vi "ERIO RT Main.vi"() -> ()   [LabVIEW 2017]
doc: "The top-level Real-Time VI for the RIO Eval Kit.\n\nThis VI runs through multiple stages. Each stage demonstrates different features of the RIO Eval Kit. The program uses a \"Queued Message Handler\" architecture. The top loop reads and writes information to and from the FPGA. That information is sent to the bottom through a queue. The information being transfered includes both the data and the type of message being sent. The bottom loop then handles displaying the appropriate information on the LCD. \n\nThe EEI IoT update to this program expands the conveyor simulation. As the encoder is moved the simulation goes through stages 1-3. When the end of 3 is met then it goes through a shutdown and back to a process reset state. At any time a shutdown, from a local source or the remote supervisor UI will put it in a reset process state. Other functions are:\n- the right button will call for an E-STOP, which will terminate the RT program\n- Alarms for signal threshold reached\n- Notifications for stage transitions and shutdown\n- Signal capture of 800 samples when triggered. \n\nInteractions are enabled by NI SystemLink, the LabVIEW Cloud Toolkit for AWS, and the LabVIEW WebVI. \n\nORIGINAL CODE: \nBy: National Instruments\n NI LabVIEW RIO Evaluation Kit\n Code example \"5- Startup Application\"\n www.ni.com/embeddedsystems\n\nUPDATED CODE: Adds NI SystemLink and NI AWS LabVIEW Tookit functionality for demonstration. \nBy: James Tillett\n Endeavor Engineering Inc.\n www.endeavoreng.com"
uses:
  <vilib>/AWS Toolkit/Core/HTTP Request/Region.ctl
  LabVIEW/Real-Time/EmbeddedDisplay/Hitachi HD44780/Common/Control/screen size.ctl
  LabVIEW/Real-Time/EmbeddedDisplay/Hitachi HD44780/Common/Control/font configuration.ctl
  LabVIEW/Controls/ERIO Queue Data.ctl
  Class EEISysLink/EEISysLink.lvclass
  LabVIEW/Controls/ERIO AWS Toolkit Variables.ctl
  <vilib>/AWS Toolkit/SQS/Queue/Queue.lvclass
  <vilib>/AWS Toolkit/SNS/Phone Number/Phone Number.lvclass
  <vilib>/AWS Toolkit/S3/Bucket/Bucket.lvclass
  LabVIEW/Controls/ERIO RT State Variables.ctl
  LabVIEW/Controls/ERIO SystemStates.ctl
  LabVIEW/Controls/ERIO Worker Variables.ctl
  LabVIEW/Controls/ERIO Globals.vi
  <vilib>/FPGAPlugInAG/sbRIO-9637/niLvFpga_Open_sbRIO-9637.vi
  <vilib>/rvi/interface/common/dynamic/niFpgaDynamicAddResources.vi
  <vilib>/Utility/error.llb/Error Cluster From Error Code.vi
  <vilib>/rvi/errors/niLvFpgaAdjustHostInterfaceError.vi
  <vilib>/FPGAPlugInAG/Dynamic/niLvFpga_Close_Dynamic.vi
  <vilib>/rvi/interface/nirviOpenFPGA/nirviOpenFPGA.xnode
  FPGA Bitfiles/ERIOLabVIEW_IoTEx_FPGATarget_FPGA_TbyGp41NgaI.lvbitx
  <vilib>/rvi/interface/nirviReadWriteControl/nirviReadWriteControl.xnode
  <vilib>/rvi/interface/nirviCloseFPGA/nirviCloseFPGA.xnode
  LabVIEW/Real-Time/EmbeddedDisplay/Hitachi HD44780/Common/HD44780 Common.lvlib
  LabVIEW/Real-Time/EmbeddedDisplay/Hitachi HD44780/Host/HD44780 Host.lvlib
  <vilib>/rvi/interface/Simulation/niFpgaSimulationCallBeginRW.vi
  NiFpgaLv.dll
  <vilib>/AWS Toolkit/Core/HTTP Request/HTTP Request.lvclass
panel:
  out "error out":errorcluster
  in  "Secret Key":string="1234567890abcdefghijklmnopqrstuvwxyz09876543221"
  out "Access Key":string
  out "Region":T1=enum."us-west-2"
  out "Phone Number":string
  out "Enable SystemLink Signal Capture":bool=TRUE
  out "Last Triggered Signal Capture":waveform(dbl)(graph)
  out "Enable S3 TDMS Signal Capture":bool=TRUE
  out "Enable SQS Notification":bool=TRUE
  out "Enable SNS Stage Notification":bool=TRUE
  out "Enable SNS Alarm Notification":bool=TRUE
  out "State":string
  out "Loop Iterations":i32
  out "Last Signal Update":waveform(dbl)(graph)
  out "Alarm":bool
  out "Alarm Threshold":dbl=4.0 format="%.3g"
  out "Amplitude":dbl format="%.3f"
  # "Start by turning encoder right to kickoff first stage, and \ncontinue turning right to complete all three stages. Stop \nthe program at any time by pressing the right button (PB2)."
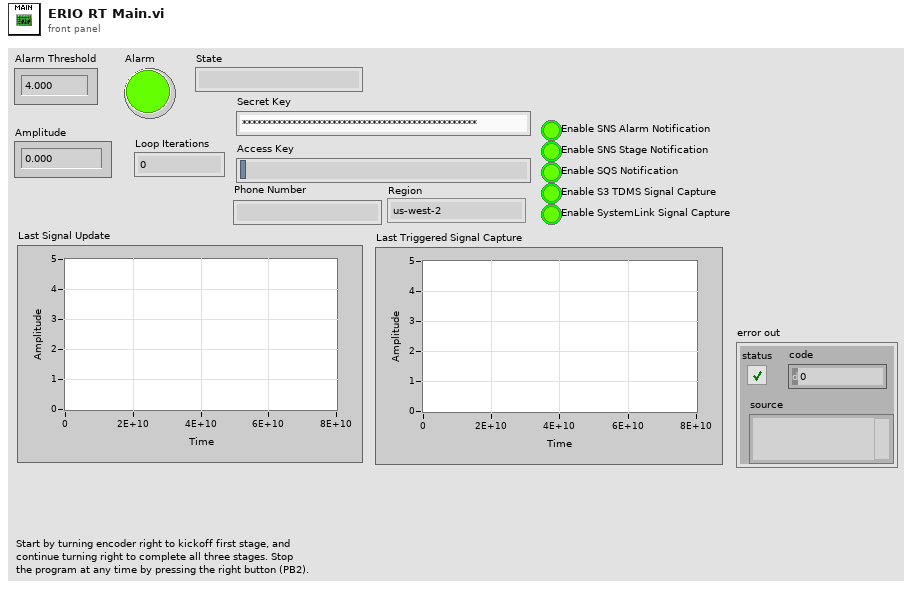
[diagram p1: front panel]
types:
  T1 = typedef "NI_AWS_Core.lvlib/HTTP Request.lvclass/Region.ctl" = enum16{"us-east-1", "us-east-2", "us-west-1", "us-west-2", "ap-northeast-1", "ap-northeast-2", "ap-southeast-1", "ap-southeast-2", "ca-central-1", "eu-central-1", "eu-west-1", "eu-west-2", "sa-east-1"}
  T2 = typedef "ERIO SystemStates.ctl" = enum16{"Shutdown", "E-STOP", "Reset Process", "Stage 1", "Stage 2", "Stage 3", "Alarm State"}
  T3 = typedef "ERIO RT State Variables.ctl" = cluster{"Position (local)":i16, "E-Stop":bool, "System State":T2, "FPGA Ref":refnum<k20>, "Previous Position (local)":i16, "Consumer Queue":refnum<queue>, "Worker Variables":T4, "Threshold Alarm":bool, "User Button":bool, "Last Signal Update":waveform(dbl)}
  T4 = typedef "ERIO Worker Variables.ctl" = cluster{"Signal Amplitude":dbl, "State":string, "Stage Percent Complete":dbl, "Alarm State":bool, "Capture Available":bool}
  T5 = typedef "ERIO AWS Toolkit Variables.ctl" = cluster{"SQS Queue":refnum<class "Queue.lvclass">, "SNS Phone Number":refnum<class "Phone Number.lvclass">, "S3 Bucket":refnum<class "Bucket.lvclass">, "SQS Init?":bool, "S3 Init?":bool, "SNS Init?":bool}
  T6 = typedef "ERIO Queue Data.ctl" = cluster{"Transition Requested":bool, "Current Pos > Previous?":bool, "Amplitude":dbl, "Stage Number":string}
  T7 = typedef "HD44780 Common.lvlib/font configuration.ctl" = enum8{"5x8 & 2 lines", "5x10 & 1 line", "5x8 & 1 line"}
  T8 = typedef "HD44780 Common.lvlib/screen size.ctl" = enum8{"8x1", "8x2", "12x4", "16x1", "16x2", "16x4", "20x1", "20x2", "20x4", "24x1", "24x2", "40x2", "40x4"}
  T9 = typedef "EEISysLink.lvclass/SL Tag Properties.ctl" = cluster{"Class Data Type":T10, "Name":string, "Description":string, "Interpolation Method":T11, "Unit of Measure":T12, "Maximum Interpolation":string, "Role":T13}
  T10 = typedef "EEISysLink.lvclass/SL Tag Data Type.ctl" = enum16{"Double", "Integer", "String", "Boolean", "Waveform"}
  T11 = typedef "EEISysLink.lvclass/SL Tag Interpolation Method.ctl" = enum16{"linear", "pilinear", "step"}
  T12 = typedef "EEISysLink.lvclass/SL Tag Unit of Measure.ctl" = enum16{"no units", "Second", "Hour", "Minute", "Day", "Year", "Month", "Week", "Foot", "Yard", "Meter", "Centimeter", "Inch", "Mile", "Nautical Mile", "Miles per Hour", "Meters per second", "Square meter", "Cubic meter", "Cubic centimeter", "Cubic inch", "Liter", "Gallon", "Gallons dry US", "Gallon UK", "Percent", "Revolutions per minute", "Revolution", "Degree angle", "Astronomical Unit", "Atom", "Atomic mass", "Bar", "Byte", "C (speed of light)", "Curie", "Decibel", "Electron Volt", "Ounce", "Knot", "G", "Grade", "Are", "Hectare", "Faraday", "Franklin", "Gilbert", "Erg", "Lambert", "Maxwell", "Gauss", "Electron mass", "Kilogram force", "Pound force", "Rad", "Centiradian", "Sphere", "Mach", "Fluid Ounces", "Fluid Ounces UK", "Fahrenheit", "Celsius", "Kelvin", "Rankine", "Gram", "Kilogram", "Pound", "Short/US Ton", "Long/UK ton", "Metric ton", "Mole", "Pounds per square inch", "Inches water column", "Torr", "Millitorr", "Millimeter mercury", "Inches mercury", "Bar (2)", "Atmosphere", "Pascal", "Watt", "kiloWatt", "Horsepower", "Kilowatt Hour", "British thermal units", "Millions of BTU", "Ampere", "Candela", "Radian", "Steradian", "Bit", "Hertz", "Newton", "Joule", "Coulomb", "Volt", "Farad", "Ohm", "Siemens", "Weber", "Tesla", "Henry", "Lumen", "Lux", "Becqueral", "Gray", "Sievert", "Katal", "Angstrom", "Light Year", "Parsec", "Point", "Pixel", "Dyne", "Kilogram force (2)", "Pound force (2)", "Rem", "Rutherford", "Roentgen"}
  T13 = typedef "EEISysLink.lvclass/SL Tag Type.ctl" = enum16{"All", "Supervisor", "Worker"}
  T14 = typedef "ERIO Supervisory Variables.ctl" = cluster{"Alarm Threshold":dbl, "Shutdown":bool, "Enable SNS Alarm":bool, "Enable SNS Stage Notification":bool, "Enable SQS Notification":bool, "Enable S3 TDMS Signal Capture":bool, "Enable SystemLink Signal Capture":bool, "Capture Signal":bool, "Server Update":bool, "AWS Access Key":string, "AWS Secret Key":string, "Phone Number":string, "Region":T1, "AWS SQS Queue":string, "AWS S3 Bucket":string}
  T15 = typedef "ERIO Alarm-Notifier Action.ctl" = enum16{"No Action", "Threshold Alarm", "Into Stage 1", "Into Stage 2", "Into Stage 3", "Into Shutdown", "Into Process Reset", "Into E-STOP", "User Button"}
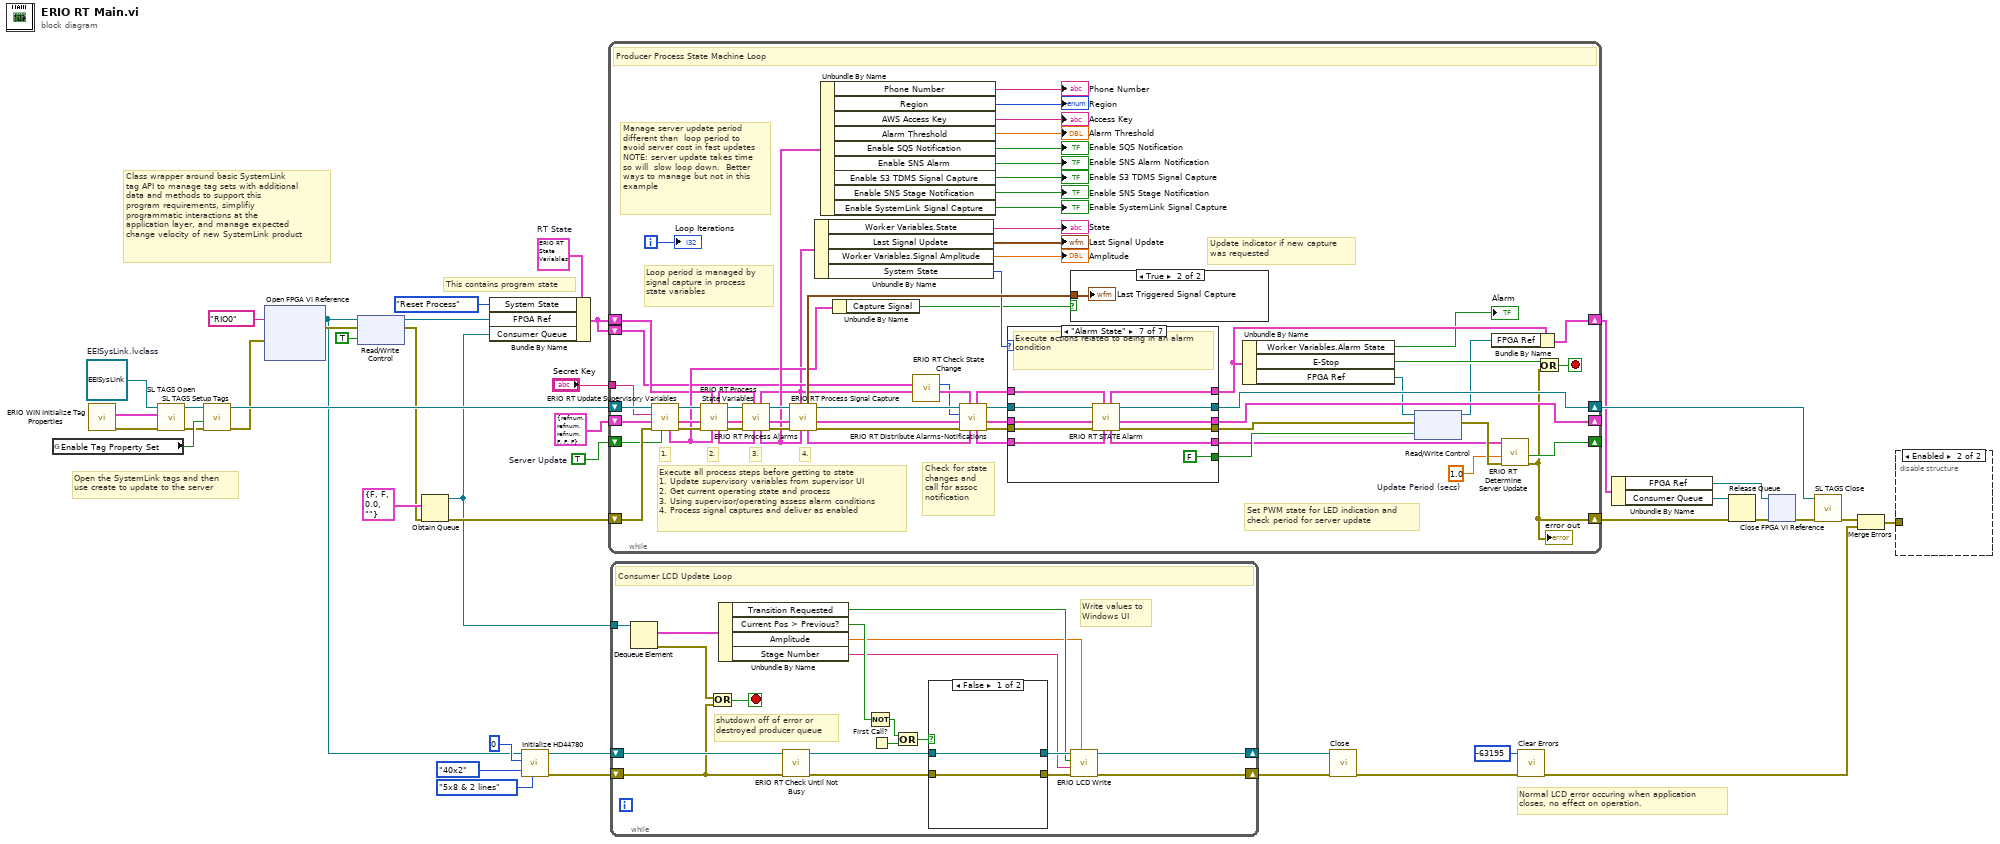
[diagram p0: block diagram]
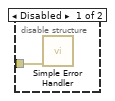
[diagram p2: hidden frame]
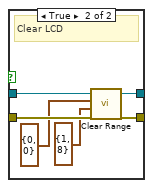
[diagram p3: hidden frame]
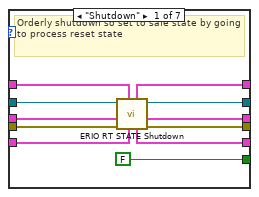
[diagram p5: hidden frame]
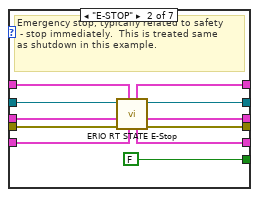
[diagram p6: hidden frame]
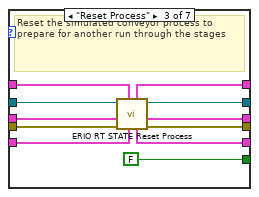
[diagram p7: hidden frame]
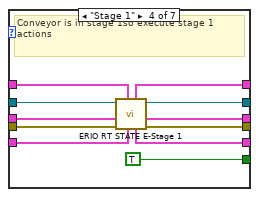
[diagram p8: hidden frame]
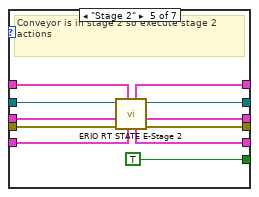
[diagram p9: hidden frame]
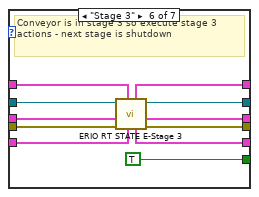
[diagram p10: hidden frame]
diagram:
  w16 = T3 {"Position (local)"=0, "E-Stop"=FALSE, "System State"=enum."Shutdown", "FPGA Ref"=refnum, "Previous Position (local)"=2, "Consumer Queue"=refnum, "Worker Variables"={"Signal Amplitude"=0.0, "State"="", "Stage Percent Complete"=0.0, "Alarm State"=FALSE, "Capture Available"=FALSE}, "Threshold Alarm"=FALSE, "User Button"=FALSE, "Last Signal Update"={"t0"=timestamp(0 s since 1904-01-01), "dt"=1.0, "Y"=[]}}  # RT State
  w20 = TRUE  # Server Update
  w23 = refnum<class "EEISysLink.lvclass"> refnum  # EEISysLink.lvclass
  # "Class wrapper around basic SystemLink\ntag API to manage tag sets with additional\ndata and methods to support this \nprogram requirements, simplifiy\nprogrammatic interactions at the \napplication layer, and manage expected\nchange velocity of new SystemLink product"
  # "This contains program state"
  # "Open the SystemLink tags and then\nuse create to update to the server"
  # "Normal LCD error occuring when application\ncloses, no effect on operation."
  n1 = global read "ERIO Globals.vi" "Enable Tag Property Set"() -> (w26:bool)
  n2 = call "ERIO WIN Initialize Tag Properties.vi"() -> ("error out"=w25:errorcluster, "Tag Properties"=w2:T9[])  [unwired: 9 in, 1 out]
  n3 = call-dynamic "SL TAGS Open.vi"("error in (no error)"=w25, "Tag Properties"=w2, "EEISysLink in"=w23) -> ("error out"=w24:errorcluster, "EEISysLink out"=w1:refnum<class "EEISysLink.lvclass">)  [unwired: 7 in]
  n4 = call-dynamic "SL TAGS Setup Tags.vi"("error in (no error)"=w24, "Set  Properties? (F)"=w26, "EEISysLink in"=w1) -> ("error out"=w22:errorcluster, "EEISysLink out"=w28:refnum<class "EEISysLink.lvclass">)  [unwired: 7 in]
  n5 = xnode ("Open FPGA VI Reference")("error in"=w22, "resource name"=tag "RIO0") -> ("FPGA VI Reference Out"=w4:refnum<k20>, "error out"=w7:errorcluster)
  n6 = xnode "Read/Write Control"("FPGA VI Reference In"=w4, "error in"=w7, "Reset"=TRUE) -> ("FPGA VI Reference Out"=w9:refnum<k20>, "error out"=w6:errorcluster)
  n7 = Obtain Queue(element data type=T6 {"Transition Requested"=FALSE, "Current Pos > Previous?"=FALSE, "Amplitude"=0.0, "Stage Number"=""} ("output to queue"), error in (no error)=w6) -> (queue out=w14:refnum<queue>, error out=w32:errorcluster)  [unwired: 3 in, 1 out]
  n8 = Bundle By Name(cluster=w16, "System State"=ERIO_SystemStates."Reset Process", "FPGA Ref"=w9, "Consumer Queue"=w14) -> (w5:T3)
  n9 = call "Initialize HD44780.vi"("font configuration (5x8 & 2 lines)"=font_configuration."5x8 & 2 lines", "screen size"=screen_size."40x2", "device index"=i8 0, "FPGA VI Reference in"=w4) -> ("error out"=w36:errorcluster, "LCD out"=w37:refnum<class "Character LCD.lvclass">)  [unwired: 6 in]
  n10 = while {
    shift-right: [w43] -> w42
    shift-left: w32 -> [w96]
    shift-right: [w73] -> w12
    shift-left: w5 -> [w62]
    shift-right: [w78] -> w18
    shift-left: w28 -> [w103]
    shift-right: [w77] -> _
    shift-left: T5 {"SQS Queue"=refnum, "SNS Phone Number"=refnum, "S3 Bucket"=refnum, "SQS Init?"=FALSE, "S3 Init?"=FALSE, "SNS Init?"=FALSE} ("AWS Variables In") -> [w102]
    shift-right: [w83] -> _
    shift-left: w20 -> [w84]
    shift-left: w5 -> [w61]
    tunnel: "Secret Key" -> [w45]
    i -> [w106]
    stop <- w97 stop-if-true
    w81 = 1.0  # Update Period (secs)
    # "4."
    # "3."
    # "2."
    # "1."
    # "Check for state\nchanges and\ncall for assoc\nnotification"
    # "Loop period is managed by\nsignal capture in process\nstate variables"
    # "Update indicator if new capture\nwas requested"
    # "Manage server update period\ndifferent than  loop period to\navoid server cost in fast updates\nNOTE: server update takes time\nso will  slow loop down.  Better\nways to manage but not in this\nexample"
    # "Set PWM state for LED indication and\ncheck period for server update"
    # "Execute all process steps before getting to state\n1. Update supervisory variables from supervisor UI\n2. Get current operating state and process\n3. Using supervisor/operating assess alarm conditions\n4. Process signal captures and deliver as enabled"
    # "Producer Process State Machine Loop"
    n11 = call "ERIO RT Update Supervisory Variables.vi"("Server Update"=w84, "error in (no error)"=w96, "AWS Variables In"=w102, "Secret Key"=w45, "EEISysLink.lvclass In"=w103) -> ("error out"=w104:errorcluster, "AWS Variables Out"=w101:T5, "EEISysLink.lvclass Out"=w105:refnum<class "EEISysLink.lvclass">, "Supervisory Variables"=w64:T14)  [unwired: 3 in]
    n12 = call "ERIO RT Process State Variables.vi"("Supervisory Variables In"=w64, "RT State In"=w62, "error in (no error)"=w104, "AWS Variables In"=w101, "EEISysLink.lvclass In"=w105) -> ("error out"=w98:errorcluster, "AWS Variables Out"=w99:T5, "EEISysLink.lvclass Out"=w100:refnum<class "EEISysLink.lvclass">, "Supervisory Variables Out"=w67:T14, "RT State Out"=w91:T3)  [unwired: 2 in]
    n13 = call "ERIO RT Process Alarms.vi"("Supervisory Variables In"=w67, "RT State In"=w91, "error in (no error)"=w98, "AWS Variables In"=w99, "EEISysLink.lvclass In"=w100) -> ("error out"=w92:errorcluster, "AWS Variables Out"=w93:T5, "EEISysLink.lvclass Out"=w94:refnum<class "EEISysLink.lvclass">, "Supervisory Variables Out"=w66:T14, "RT State Out"=w60:T3)  [unwired: 2 in]
    n14 = call "ERIO RT Process Signal Capture.vi"("Supervisory Variables In"=w66, "RT State"=w60, "error in (no error)"=w92, "AWS Variables In"=w93, "EEISysLink.lvclass In"=w94) -> ("error out"=w56:errorcluster, "AWS Variables Out"=w57:T5, "EEISysLink.lvclass Out"=w59:refnum<class "EEISysLink.lvclass">, "Supervisory Variables Out"=w51:T14, "Last Triggered Signal Capture"=w90:waveform(dbl))  [unwired: 2 in]
    n15 = Unbundle By Name(w60) -> ("Worker Variables.State"=→"State":string, "Last Signal Update"=→"Last Signal Update":waveform(dbl), "Worker Variables.Signal Amplitude"=→"Amplitude":dbl, "System State"=w65:T2)
    n16 = Unbundle By Name(w66) -> ("Phone Number"=→"Phone Number":string, "Region"=→"Region":T1, "AWS Access Key"=→"Access Key":string, "Alarm Threshold"=→"Alarm Threshold":dbl, "Enable SQS Notification"=→"Enable SQS Notification":bool, "Enable SNS Alarm"=→"Enable SNS Alarm Notification":bool, "Enable S3 TDMS Signal Capture"=→"Enable S3 TDMS Signal Capture":bool, "Enable SNS Stage Notification"=→"Enable SNS Stage Notification":bool, "Enable SystemLink Signal Capture"=→"Enable SystemLink Signal Capture":bool)
    n17 = Unbundle By Name(w64) -> ("Capture Signal"=w63:bool)
    n18 = call "ERIO RT Check State Change.vi"("RT Current State In"=w60, "RT Previous State"=w61) -> ("RT Current State Out"=w53:T3, "Alarm-Notifier Action"=w49:T15)  [unwired: 8 in]
    n19 = call "ERIO RT Distribute Alarms-Notifications.vi"("Supervisory Variables In"=w51, "RT State In"=w53, "error in (no error)"=w56, "AWS Variables In"=w57, "Alarm-Notifier"=w49, "EEISysLink.lvclass In"=w59) -> ("error out"=w55:errorcluster, "AWS Variables Out"=w54:T5, "EEISysLink.lvclass Out"=w58:refnum<class "EEISysLink.lvclass">, "Supervisory Variables Out"=w50:T14, "RT State Out"=w52:T3)  [unwired: 1 in]
    n20 = case shown="\"Alarm State\"" w65 {
      tunnel: w55 -> [w115 w125 w136 w147 w161 w172 w175]
      tunnel: [FALSE FALSE FALSE TRUE ("PWM") TRUE ("PWM") TRUE ("PWM") FALSE] -> w86
      tunnel: w58 -> [w117 w122 w133 w150 w158 w171 w177]
      tunnel: w54 -> [w116 w126 w137 w148 w157 w170 w176]
      tunnel: w52 -> [w112 w128 w139 w143 w160 w168 w178]
      tunnel: w50 -> [w114 w120 w131 w142 w153 w164 w174]
      tunnel: [w113 w121 w132 w149 w154 w166 w183] -> w78
      tunnel: [w108 w127 w138 w144 w159 w167 w180] -> w75
      tunnel: [w111 w123 w134 w145 w155 w165 w181] -> w77
      tunnel: [w110 w124 w135 w146 w156 w169 w182] -> w80
      tunnel: [w109 w119 w130 w141 w152 w163 w179] -> w79
      frame "Shutdown" {
        # "Orderly shutdown so set to safe state by going to process reset state"
        n21 = call "ERIO RT STATE Shutdown.vi"("Supervisory Variables In"=w114, "RT State In"=w112, "error in (no error)"=w115, "AWS Variables In"=w116, "EEISysLink.lvclass In"=w117) -> ("error out"=w110:errorcluster, "AWS Variables Out"=w111:T5, "EEISysLink.lvclass Out"=w113:refnum<class "EEISysLink.lvclass">, "Supervisory Variables Out"=w109:T14, "RT State Out"=w108:T3)  [unwired: 2 in]
      }
      frame "E-STOP" {
        # "Emergency stop, typically related to safety\n - stop immediately.  This is treated same\nas shutdown in this example."
        n22 = call "ERIO RT STATE E-Stop.vi"("Supervisory Variables In"=w120, "RT State In"=w128, "error in (no error)"=w125, "AWS Variables In"=w126, "EEISysLink.lvclass In"=w122) -> ("error out"=w124:errorcluster, "AWS Variables Out"=w123:T5, "EEISysLink.lvclass Out"=w121:refnum<class "EEISysLink.lvclass">, "Supervisory Variables Out"=w119:T14, "RT State Out"=w127:T3)  [unwired: 2 in]
      }
      frame "Reset Process" {
        # "Reset the simulated conveyor process to prepare for another run through the stages"
        n23 = call "ERIO RT STATE Reset Process.vi"("Supervisory Variables In"=w131, "RT State In"=w139, "error in (no error)"=w136, "AWS Variables In"=w137, "EEISysLink.lvclass In"=w133) -> ("error out"=w135:errorcluster, "AWS Variables Out"=w134:T5, "EEISysLink.lvclass Out"=w132:refnum<class "EEISysLink.lvclass">, "Supervisory Variables Out"=w130:T14, "RT State Out"=w138:T3)  [unwired: 2 in]
      }
      frame "Stage 1" {
        # "Conveyor is in stage 1so execute stage 1\nactions"
        n24 = call "ERIO RT STATE E-Stage 1.vi"("Supervisory Variables In"=w142, "RT State In"=w143, "error in (no error)"=w147, "AWS Variables In"=w148, "EEISysLink.lvclass In"=w150) -> ("error out"=w146:errorcluster, "AWS Variables Out"=w145:T5, "EEISysLink.lvclass Out"=w149:refnum<class "EEISysLink.lvclass">, "Supervisory Variables Out"=w141:T14, "RT State Out"=w144:T3)  [unwired: 2 in]
      }
      frame "Stage 2" {
        # "Conveyor is in stage 2 so execute stage 2\nactions"
        n25 = call "ERIO RT STATE E-Stage 2.vi"("Supervisory Variables In"=w153, "RT State In"=w160, "error in (no error)"=w161, "AWS Variables In"=w157, "EEISysLink.lvclass In"=w158) -> ("error out"=w156:errorcluster, "AWS Variables Out"=w155:T5, "EEISysLink.lvclass Out"=w154:refnum<class "EEISysLink.lvclass">, "Supervisory Variables Out"=w152:T14, "RT State Out"=w159:T3)  [unwired: 2 in]
      }
      frame "Stage 3" {
        # "Conveyor is in stage 3 so execute stage 3\nactions - next stage is shutdown"
        n26 = call "ERIO RT STATE E-Stage 3.vi"("Supervisory Variables In"=w164, "RT State In"=w168, "error in (no error)"=w172, "AWS Variables In"=w170, "EEISysLink.lvclass In"=w171) -> ("error out"=w169:errorcluster, "AWS Variables Out"=w165:T5, "EEISysLink.lvclass Out"=w166:refnum<class "EEISysLink.lvclass">, "Supervisory Variables Out"=w163:T14, "RT State Out"=w167:T3)  [unwired: 2 in]
      }
      frame "Alarm State" {
        # "Execute actions related to being in an alarm condition"
        n27 = call "ERIO RT STATE Alarm.vi"("Supervisory Variables In"=w174, "RT State In"=w178, "error in (no error)"=w175, "AWS Variables In"=w176, "EEISysLink.lvclass In"=w177) -> ("error out"=w182:errorcluster, "AWS Variables Out"=w181:T5, "EEISysLink.lvclass Out"=w183:refnum<class "EEISysLink.lvclass">, "Supervisory Variables Out"=w179:T14, "RT State Out"=w180:T3)  [unwired: 2 in]
      }
    }
    n28 = case shown="True" w63 {
      tunnel: w90 -> [_ w107]
      frame False {
      }
      frame True {
        "Last Triggered Signal Capture" <- w107
      }
    }
    n29 = Unbundle By Name(w75) -> ("Worker Variables.Alarm State"=→"Alarm":bool, "E-Stop"=w85:bool, "FPGA Ref"=w76:refnum<k20>)
    n30 = xnode ("Read/Write Control")("FPGA VI Reference In"=w76, "error in"=w80, "PWM"=w86) -> ("FPGA VI Reference Out"=w74:refnum<k20>, "error out"=w82:errorcluster)
    n31 = Bundle By Name(cluster=w75, "FPGA Ref"=w74) -> (w73:T3)
    n32 = call "ERIO RT Determine Server Update.vi"("error in (no error)"=w82, "Update Period (secs)"=w81, "Supervisory Variables In"=w79) -> ("error out"=w43:errorcluster, "Update Server"=w83:bool)  [unwired: 6 in, 1 out]
    "error out" <- w43
    n33 = Or(x=w85, y=w43) -> (x .or. y?=w97:bool)
    "Loop Iterations" <- w106
  }
  n34 = while {
    shift-right: [w193] -> w35
    shift-left: w37 -> [w203]
    shift-right: [w190] -> w34
    shift-left: w36 -> [w202]
    tunnel: w14 -> [w201]
    stop <- w192 stop-if-true
    # "Write values to\nWindows UI"
    # "shutdown off of error or \ndestroyed producer queue"
    # "Consumer LCD Update Loop"
    n35 = Dequeue Element(queue=w201) -> (element=w189:T6, error out=w200:errorcluster)  [unwired: 2 in, 2 out]
    n36 = Or(x=w200, y=w202) -> (x .or. y?=w192:bool)
    n37 = Unbundle By Name(w189) -> ("Transition Requested"=w188:bool, "Current Pos > Previous?"=w187:bool, "Amplitude"=w185:dbl, "Stage Number"=w186:string)
    n38 = call "ERIO RT Check Until Not Busy.vi"("error in"=w202, "LCD in"=w203) -> ("error out"=w191:errorcluster, "LCD out"=w199:refnum<class "Character LCD.lvclass">)  [unwired: 8 in]
    n39 = Not(x=w187) -> (.not. x?=w194:bool)
    n40 = First Call?() -> (First Call?: T/F=w195:bool)
    n41 = Or(x=w194, y=w195) -> (x .or. y?=w196:bool)
    n42 = case shown="False" w196 {
      tunnel: w199 -> [w205 w211]
      tunnel: w191 -> [w204 w210]
      tunnel: [w204 w209] -> w197
      tunnel: [w205 w208] -> w198
      frame False {
      }
      frame True {
        # "Clear LCD"
        n43 = call "Clear Range.vi"("error in (no error)"=w210, "end position (end of line)"=cluster{"row":i8, "column":i8} {"row"=1, "column"=8} ("start position"), "start position"=cluster{"row":i8, "column":i8} {"row"=0, "column"=0}, "LCD in"=w211) -> ("error out"=w209:errorcluster, "LCD out"=w208:refnum<class "Character LCD.lvclass">)  [unwired: 6 in]
      }
    }
    n44 = call "ERIO LCD Write.vi"("Amplitude"=w185, "error in (no error)"=w197, "Stage Number"=w186, "Current Pos > Threshold?"=w188, "Character LCD in"=w198) -> ("error out"=w190:errorcluster, "LCD out"=w193:refnum<class "Character LCD.lvclass">)  [unwired: 4 in]
  }
  n45 = call "Close.vi"("error in (no error)"=w34, "LCD in"=w35) -> ("error out"=w29:errorcluster)  [unwired: 9 in]
  n46 = call <vilib>:"Clear Errors.vi"("error in (no error)"=w29, "specific error code to clear (0: all)"=-63195) -> ("error out"=w31:errorcluster)  [unwired: 4 in, 1 out]
  n47 = Unbundle By Name(w12) -> ("FPGA Ref"=w10:refnum<k20>, "Consumer Queue"=w11:refnum<queue>)
  n48 = Release Queue(queue=w11, error in (no error)=w42) -> (error out=w41:errorcluster)  [unwired: 1 in, 2 out]
  n49 = xnode "Close FPGA VI Reference"("FPGA VI Reference In"=w10, "error in"=w41) -> ("error out"=w19:errorcluster)
  n50 = call-dynamic "SL TAGS Close.vi"("error in (no error)"=w19, "EEISysLink in"=w18) -> ("error out"=w17:errorcluster)  [unwired: 8 in, 1 out]
  n51 = Merge Errors(w17, w31) -> (w33:errorcluster)
  n52 = disable-structure shown="Enabled" {
    disable-tunnel: w33 -> [w212 _]
    frame Disabled {
      n53 = call <vilib>:"Simple Error Handler.vi"("error in (no error)"=w212) -> ()  [unwired: 4 in, 5 out]
    }
    frame Enabled {
    }
  }
